vi "GetItemNames.vi"(9 "AnalysisResultNum":i32, 10 "FilteredCaliperEntry":T6[](array[typedef]) {"CaliperType" items=["Distance", "Mid Point", "Perpendicular Projection", "Lines Intersection", "Angle from Horizontal", "Angle from Vertical", "Angle Defined by 3 Points", "Angle Defined by 4 Points", "Bissecting Line", "Mid Line", "Center of Mass", "Area", "Line Fit", "Circle Fit", "Ellipse Fit"]}, 11 "Item Names":string[][](array[string])) -> (2 "NameTagToAdd":string[](array[string]), 3 "Action":enum16{"None", "Add", "Delete"}(ring))   [LabVIEW 2019]
uses:
  Controls/CaliperDataEntry_SinglePoint.ctl
  Controls/CaliperType.ctl
  Controls/SelectionListEntry.ctl
  Controls/SelectionListEntryPointType.ctl
  Controls/CaliperResult_SinglePoint.ctl
  Controls/CaliperDataEntry.ctl
  Controls/CaliperResult.ctl
panel:
  in  "CaliperEntry":T1 {"CaliperType" items=["Distance", "Mid Point", "Perpendicular Projection", "Lines Intersection", "Angle from Horizontal", "Angle from Vertical", "Angle Defined by 3 Points", "Angle Defined by 4 Points", "Bissecting Line", "Mid Line", "Center of Mass", "Area", "Line Fit", "Circle Fit", "Ellipse Fit"]}
  out "EqualNum?":bool
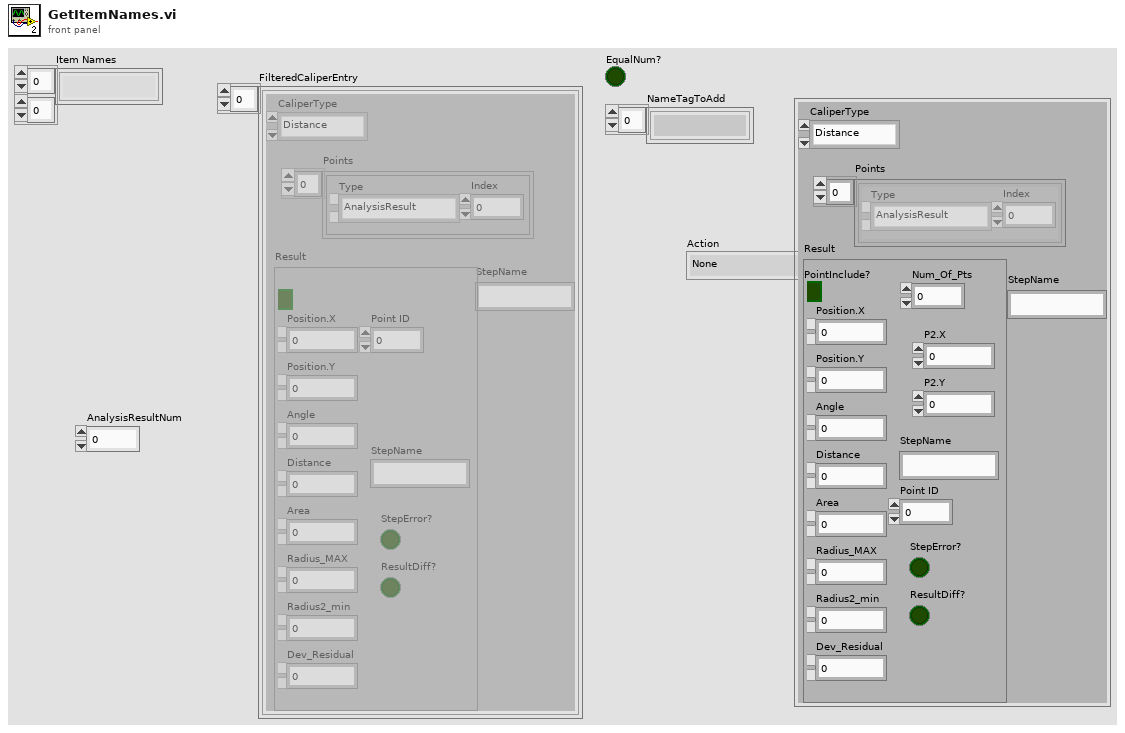
[diagram p1: front panel]
types:
  T1 = typedef "CaliperDataEntry.ctl" = cluster{"CaliperType":T2, "Points":T3[], "Result":T5, "StepName":string}
  T2 = typedef "CaliperType.ctl" = u32
  T3 = typedef "SelectionListEntry.ctl" = cluster{"Type":T4, "Index":i32}
  T4 = typedef "SelectionListEntryPointType.ctl" = enum16{"AnalysisResult", "CaliperResult"}
  T5 = typedef "CaliperResult.ctl" = cluster{"PointInclude?":bool, "Num_Of_Pts":u8, "Position.X":dbl, "Position.Y":dbl, "Angle":dbl, "Distance":dbl, "Area":dbl, "Radius_MAX":dbl, "Radius2_min":dbl, "Dev_Residual":dbl, "P2.X":dbl, "P2.Y":dbl, "StepName":string, "Point ID":u8, "StepError?":bool, "ResultDiff?":bool}
  T6 = typedef "CaliperDataEntry_SinglePoint.ctl" = cluster{"CaliperType":T2, "Points":T3[], "Result":T7, "StepName":string}
  T7 = typedef "CaliperResult_SinglePoint.ctl" = cluster{"PointInclude?":bool, "Position.X":dbl, "Position.Y":dbl, "Angle":dbl, "Distance":dbl, "Area":dbl, "Radius_MAX":dbl, "Radius2_min":dbl, "Dev_Residual":dbl, "StepName":string, "Point ID":u8, "StepError?":bool, "ResultDiff?":bool}
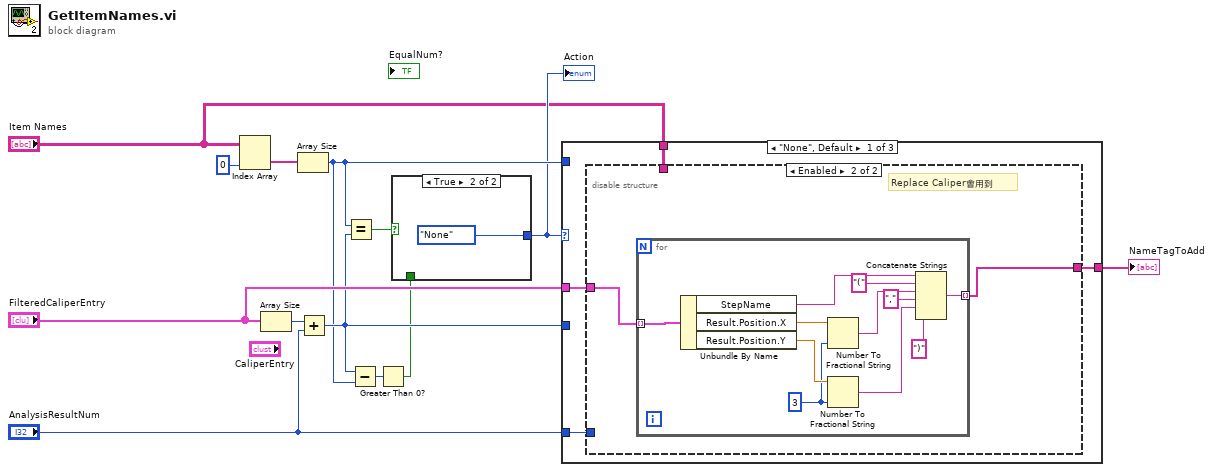
[diagram p0: block diagram]
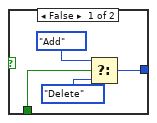
[diagram p2: hidden frame]
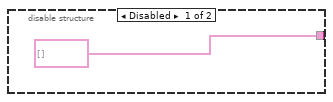
[diagram p3: hidden frame]
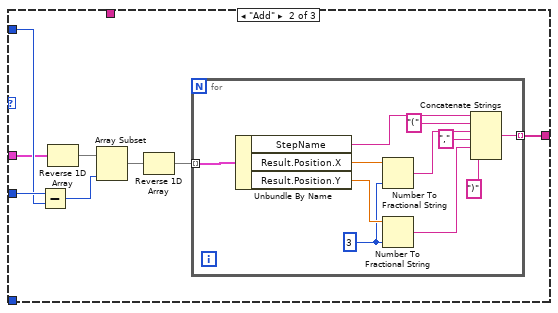
[diagram p4: hidden frame]
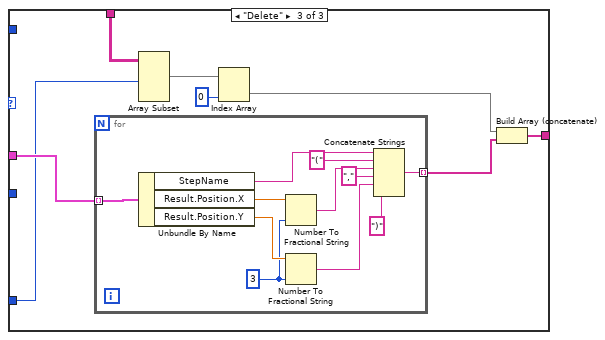
[diagram p5: hidden frame]
diagram:
  n1 = Index Array(array="Item Names", index (col)=0 ("disabled index (col)")) -> (element=w11:string[])  [unwired: 1 in]
  n2 = Array Size(array="FilteredCaliperEntry") -> (size(s)=w13:i32)
  n3 = Array Size(array=w11) -> (size(s)=w6:i32)
  n4 = Add(x=w13, y="AnalysisResultNum") -> (x+y=w7:i32)
  n5 = Equal?(x=w6, y=w7) -> (x = y?=w8:bool)
  n6 = Subtract(x=w7, y=w6) -> (x-y=w5:i32)
  n7 = Greater Than 0?(x=w5) -> (x > 0?=w4:bool)
  n8 = case shown="True" w8 {
    tunnel: [w17 enum16{"None", "Add", "Delete"}."None" ("Action")] -> w3
    tunnel: w4 -> [w16 _]
    frame False {
      n9 = Select(t=enum16{"None", "Add", "Delete"}."Add" ("Action"), s=w16, f=enum16{"None", "Add", "Delete"}."Delete" ("Action")) -> (s? t:f=w17:enum16{"None", "Add", "Delete"})
    }
    frame True {
    }
  }
  "Action" <- w3
  n10 = case shown="\"None\", Default" w3 {
    tunnel: w7 -> [_ w44 _]
    tunnel: w6 -> [_ w43 _]
    tunnel: "FilteredCaliperEntry" -> [w19 w42 w63]
    tunnel: [w22 w37 w61] -> w9
    tunnel: "Item Names" -> [w21 _ w60]
    tunnel: "AnalysisResultNum" -> [w20 _ w59]
    frame "None", Default {
      n11 = disable-structure shown="Enabled" {
        disable-tunnel: [string[] [] w24] -> w22
        disable-tunnel: w21 -> [_ _]
        disable-tunnel: w20 -> [_ _]
        disable-tunnel: w19 -> [_ w25]
        frame Disabled {
        }
        frame Enabled {
          # "Replace Caliper會用到"
          n12 = for {
            tunnel: w25 -> [w36] mode=indexing
            tunnel: [w26] -> w24 mode=indexing
            w31 = i16 3 ("precision (6)")
            n13 = Unbundle By Name(w36) -> ("StepName"=w35:string, "Result.Position.X"=w33:dbl, "Result.Position.Y"=w32:dbl)
            n14 = Number To Fractional String(number=w33, precision (6)=w31) -> (F-format string=w30:string)  [unwired: 2 in]
            n15 = Number To Fractional String(number=w32, precision (6)=w31) -> (F-format string=w29:string)  [unwired: 2 in]
            n16 = Concatenate Strings(w35, "(" ("string"), w30, "," ("string"), w29, ")" ("string")) -> (w26:string)
          }
        }
      }
    }
    frame "Add" {
      n17 = Subtract(x=w44, y=w43) -> (x-y=w40:i32)
      n18 = Reverse 1D Array(array=w42) -> (reversed array=w41:T6[])
      n19 = Array Subset(array=w41, length=w40) -> (w39:T6[])  [unwired: 1 in]
      n20 = Reverse 1D Array(array=w39) -> (reversed array=w38:T6[])
      n21 = for {
        tunnel: w38 -> [w55] mode=indexing
        tunnel: [w45] -> w37 mode=indexing
        w50 = i16 3 ("precision (6)")
        n22 = Unbundle By Name(w55) -> ("StepName"=w54:string, "Result.Position.X"=w52:dbl, "Result.Position.Y"=w51:dbl)
        n23 = Number To Fractional String(number=w52, precision (6)=w50) -> (F-format string=w49:string)  [unwired: 2 in]
        n24 = Number To Fractional String(number=w51, precision (6)=w50) -> (F-format string=w48:string)  [unwired: 2 in]
        n25 = Concatenate Strings(w54, "(" ("string"), w49, "," ("string"), w48, ")" ("string")) -> (w45:string)
      }
    }
    frame "Delete" {
      n26 = for {
        tunnel: w63 -> [w74] mode=indexing
        tunnel: [w64] -> w62 mode=indexing
        w69 = i16 3 ("precision (6)")
        n27 = Unbundle By Name(w74) -> ("StepName"=w73:string, "Result.Position.X"=w71:dbl, "Result.Position.Y"=w70:dbl)
        n28 = Number To Fractional String(number=w71, precision (6)=w69) -> (F-format string=w68:string)  [unwired: 2 in]
        n29 = Number To Fractional String(number=w70, precision (6)=w69) -> (F-format string=w67:string)  [unwired: 2 in]
        n30 = Concatenate Strings(w73, "(" ("string"), w68, "," ("string"), w67, ")" ("string")) -> (w64:string)
      }
      n31 = Array Subset(array=w60, length (row)=w59) -> (w57:string[][])  [unwired: 3 in]
      n32 = Index Array(array=w57, index (col)=0 ("disabled index (col)")) -> (element=w56:string[])  [unwired: 1 in]
      n33 = Build Array (concatenate)(w56, w62) -> (w61:string[])
    }
  }
  "NameTagToAdd" <- w9
